vi "Axsun_subvi.vi"(10 "Clock delay":u32, 11 "Action":T1) -> (0 "error out":errorcluster, 3 "output cluster":T2)   [LabVIEW 2018]
uses:
  cluster_Axsun.ctl
  Action_Axsun.ctl
  C:/Users/BoasLab/Documents/stephan/Axsun control/AxsunOCTControl.dll
  AxsunOCTControl.dll
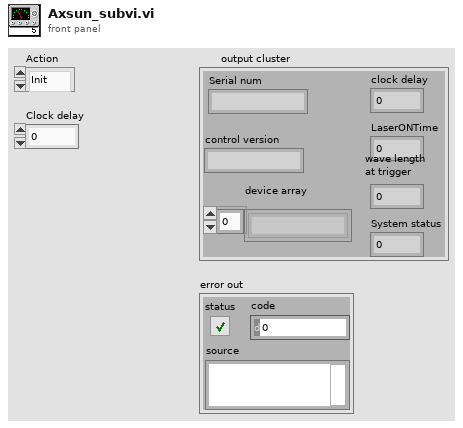
[diagram p1: front panel]
types:
  T1 = typedef "Action_Axsun.ctl" = enum16{"Init", "Stop", "Source current ON", "Source current OFF", "Laser ON", "Laser OFF", "GetLaserOnTime", "Clock delay"}
  T2 = typedef "cluster_Axsun.ctl" = cluster{"device array":string[], "control version":string, "Serial num":string, "LaserONTime":i32, "wave length\nat trigger":dbl, "System status":dbl, "clock delay":u32}
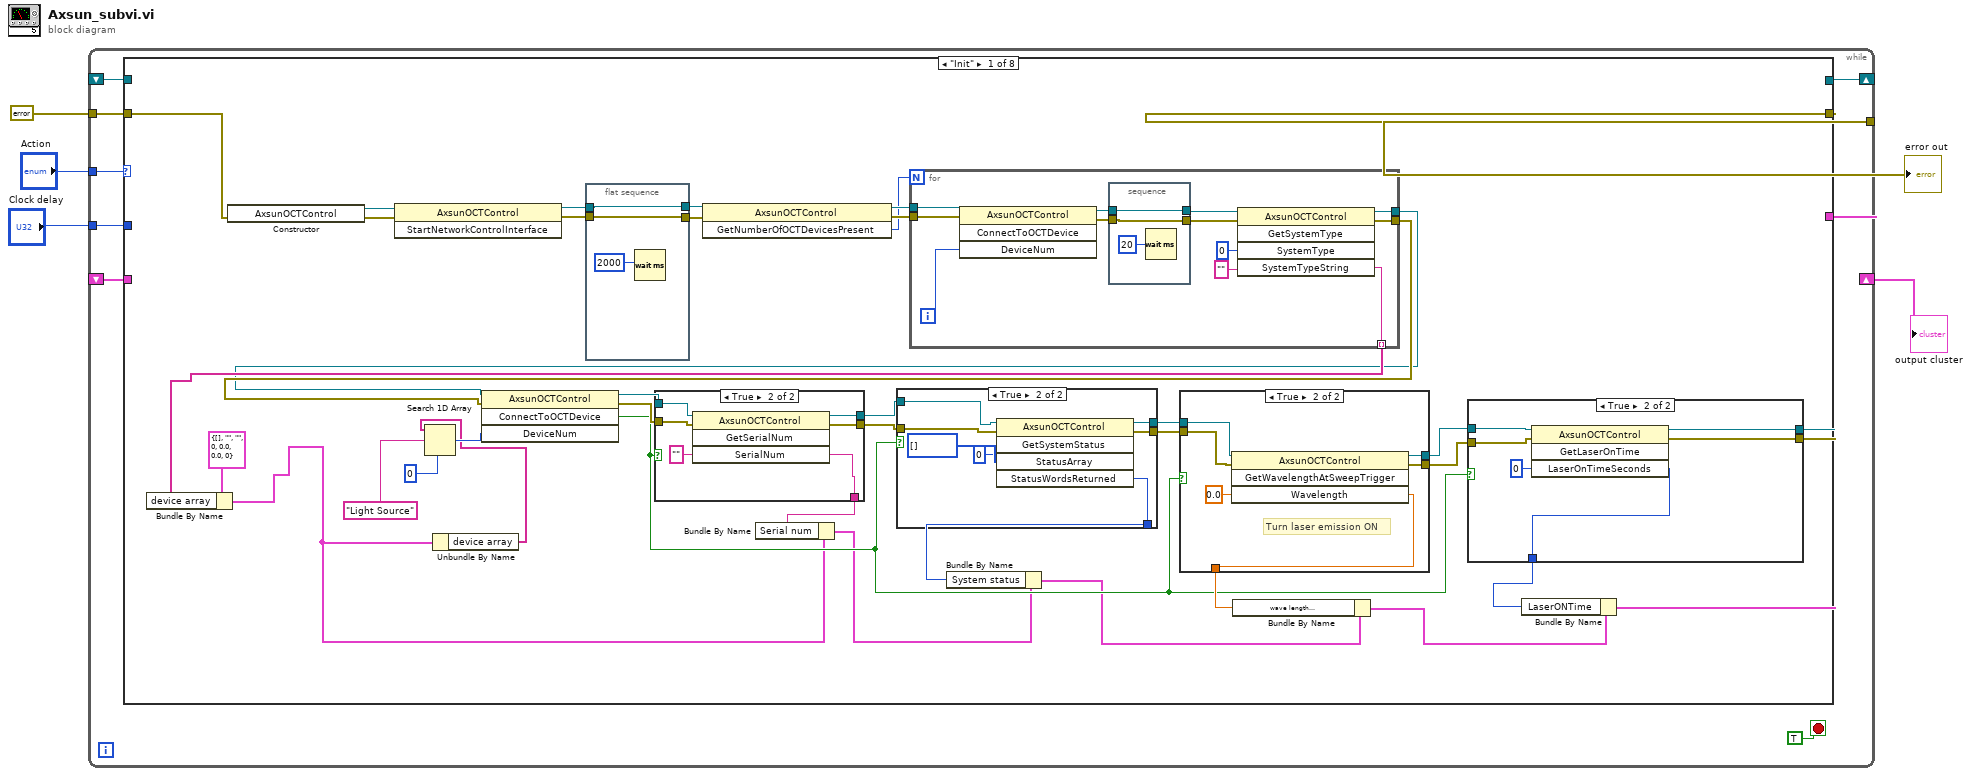
[diagram p0: block diagram]
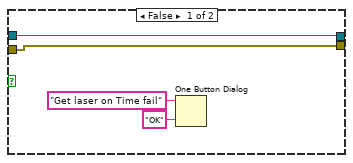
[diagram p2: hidden frame]
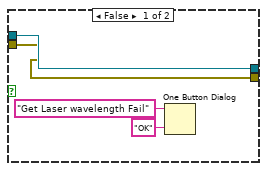
[diagram p3: hidden frame]
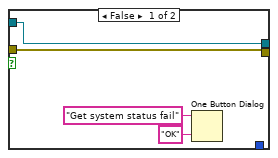
[diagram p4: hidden frame]
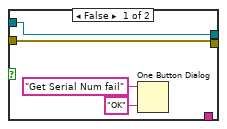
[diagram p5: hidden frame]
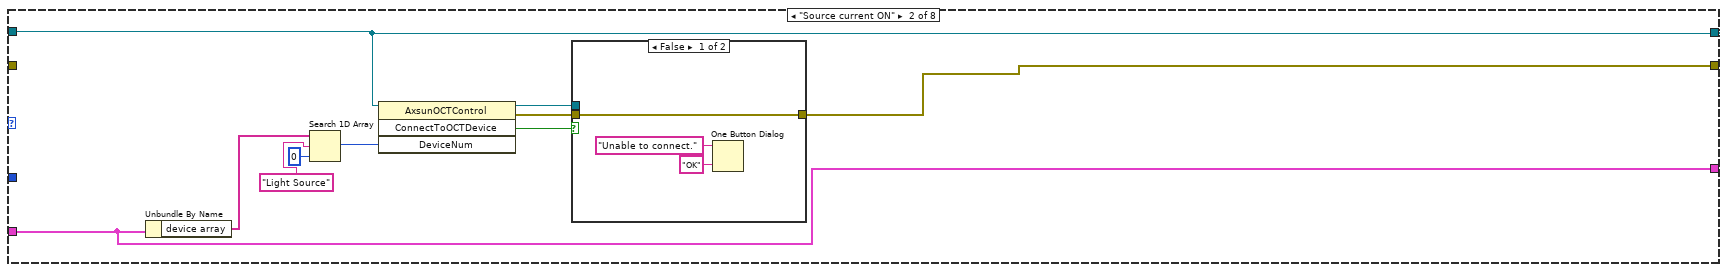
[diagram p6: hidden frame]
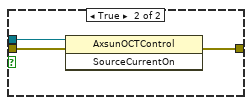
[diagram p7: hidden frame]
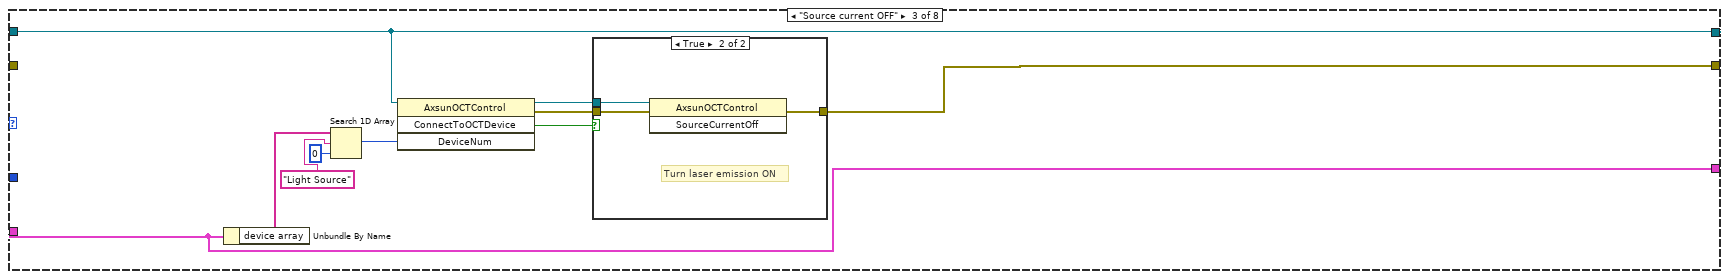
[diagram p8: hidden frame]
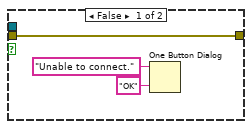
[diagram p9: hidden frame]
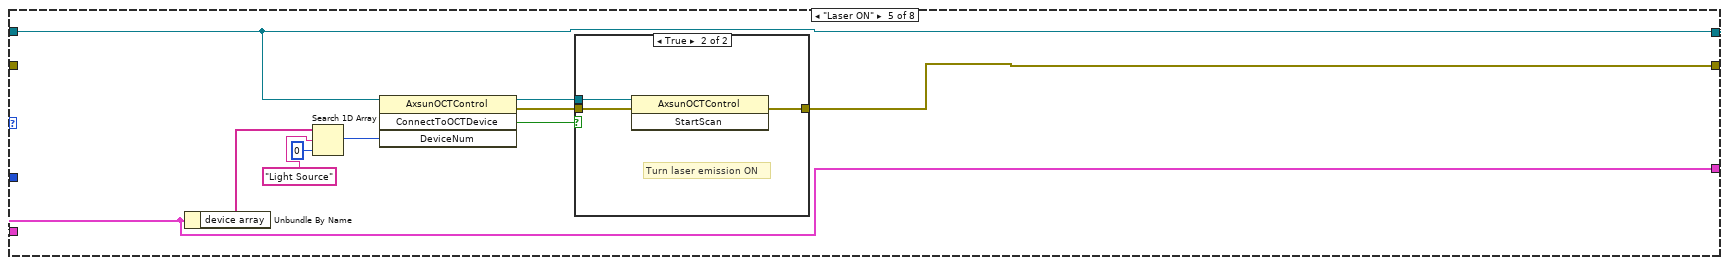
[diagram p11: hidden frame]
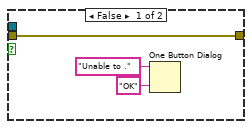
[diagram p12: hidden frame]
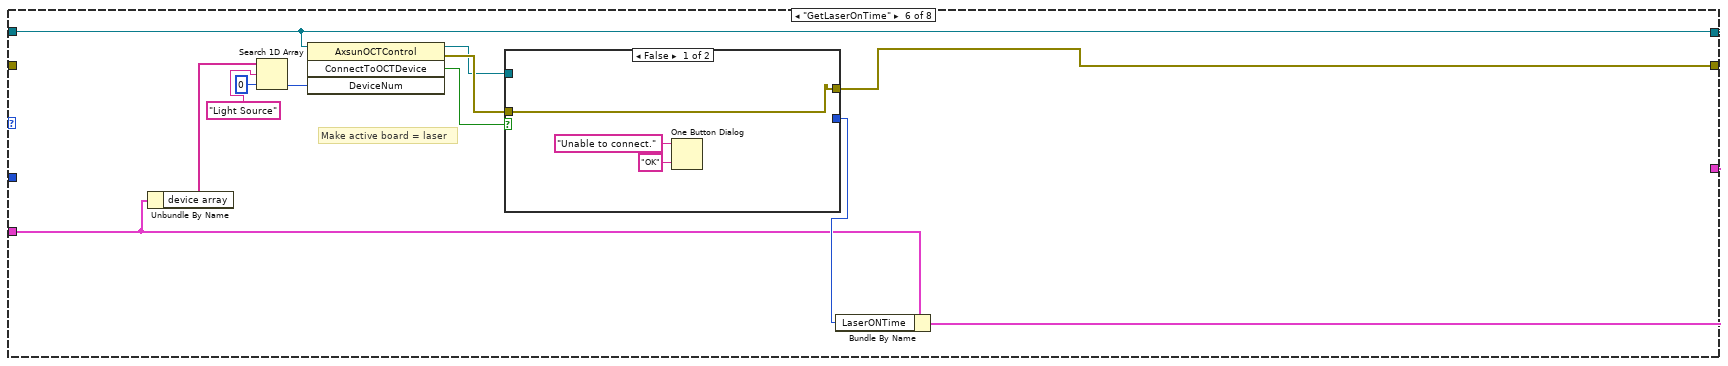
[diagram p13: hidden frame]
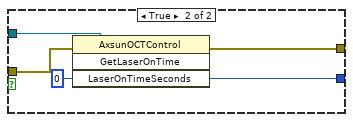
[diagram p14: hidden frame]
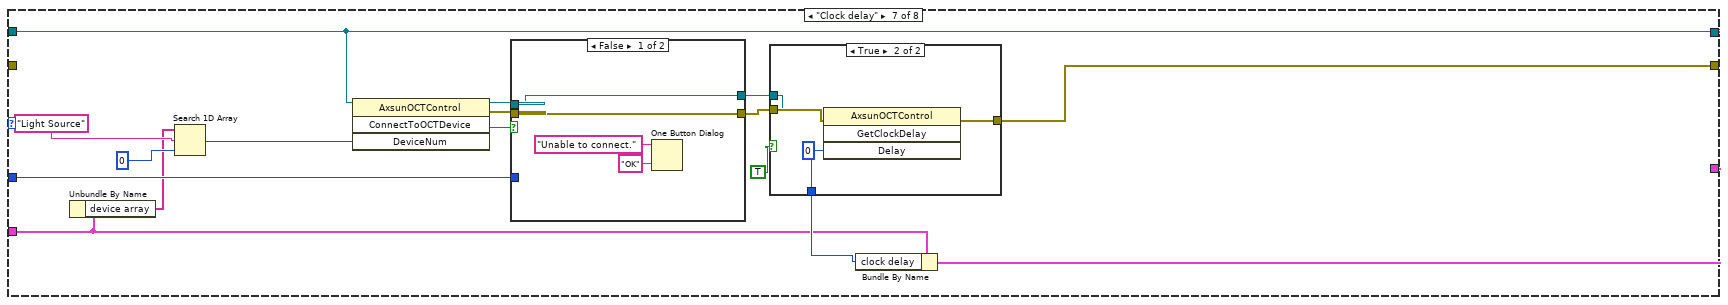
[diagram p15: hidden frame]
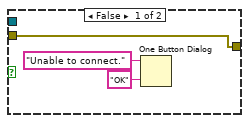
[diagram p16: hidden frame]
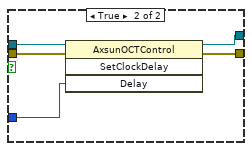
[diagram p17: hidden frame]
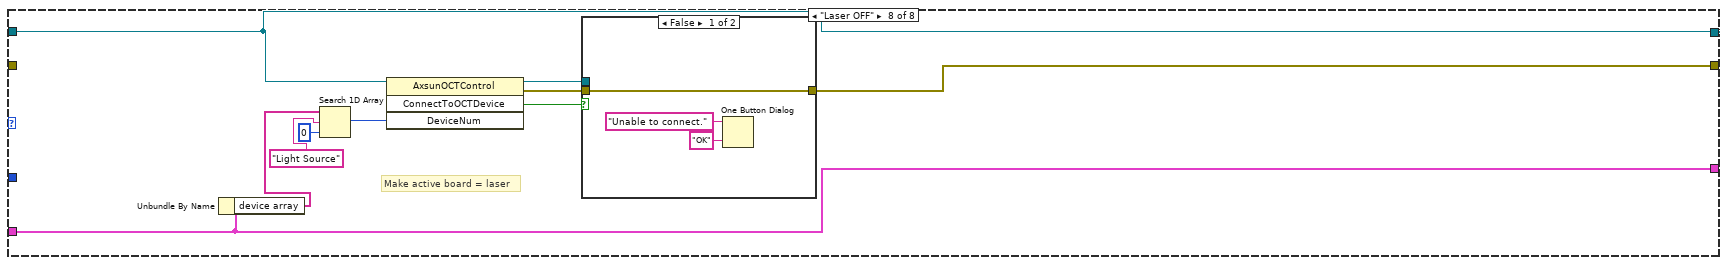
[diagram p18: hidden frame]
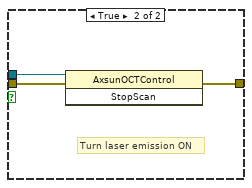
[diagram p19: hidden frame]
diagram:
  n1 = while {
    shift-right: [w11] -> _
    shift-left: _ -> [w12]
    shift-right: [w8] -> w2
    shift-left: _ -> [w14]
    tunnel: [w13] -> w4
    tunnel: "Clock delay" -> [w10]
    tunnel: "Action" -> [w9]
    tunnel: errorcluster {"status"=FALSE, "code"=0, "source"=""} ("error in (no error)") -> [w6]
    stop <- TRUE ("stop") stop-if-true
    n2 = case shown="\"Init\"" w9 {
      tunnel: [w28 w116 w132 _ w150 w168 w190 w219] -> w13
      tunnel: [w24 w113 w129 w144 w147 w163 w187 w216] -> w8
      tunnel: w14 -> [_ w113 w129 w144 w147 w166 w185 w216]
      tunnel: [w29 w112 w128 w145 w146 w162 w183 w215] -> w11
      tunnel: w12 -> [_ w112 w128 w145 w146 w162 w183 w215]
      tunnel: w10 -> [_ _ _ _ _ _ w188 _]
      tunnel: w6 -> [w15 _ _ _ _ _ _ _]
      frame "Init" {
        n3 = constructor class="AxsunOCTControl"(error in=w15) -> (reference out=w52:refnum<k24>, error out=w51:errorcluster)  [unwired: 2 in, 1 out]
        n4 = invoke class="AxsunOCTControl" method="StartNetworkControlInterface"(reference=w52, error in=w51) -> (reference out=w50:refnum<k24>, error out=w48:errorcluster)  [unwired: 1 in, 1 out]
        n5 = flat-sequence {
          tunnel: w50 -> [w110]
          tunnel: [w110] -> w49
          tunnel: [w109] -> w47
          tunnel: w48 -> [w109]
          frame #0 {
            n6 = Wait (ms)(milliseconds to wait=2000) -> ()  [unwired: 1 out]
          }
        }
        n7 = invoke class="AxsunOCTControl" method="GetNumberOfOCTDevicesPresent"(reference=w49, error in=w47) -> (reference out=w46:refnum<k24>, error out=w45:errorcluster, "GetNumberOfOCTDevicesPresent"=w19:i32)  [unwired: 1 in]
        n8 = for {
          N: w19 -> [_]
          tunnel: [w98] -> w18
          tunnel: [w97] -> w17
          tunnel: w46 -> [w96]
          tunnel: w45 -> [w95]
          tunnel: [w94] -> w23 mode=indexing
          i -> [w99]
          n9 = invoke class="AxsunOCTControl" method="ConnectToOCTDevice"(reference=w96, error in=w95, "DeviceNum"=w99) -> (reference out=w103:refnum<k24>, error out=w102:errorcluster)  [unwired: 1 in, 2 out]
          n10 = stacked-sequence {
            tunnel: w103 -> [w108]
            tunnel: [w108] -> w101
            tunnel: w102 -> [w107]
            tunnel: [w107] -> w100
            frame #0 {
              n11 = Wait (ms)(milliseconds to wait=u32 20) -> ()  [unwired: 1 out]
            }
          }
          n12 = invoke class="AxsunOCTControl" method="GetSystemType"(reference=w101, error in=w100, "SystemType"=u32 0, "SystemTypeString"="") -> (reference out=w97:refnum<k24>, error out=w98:errorcluster, "SystemTypeString"=w94:string)  [unwired: 1 in, 2 out]
        }
        n13 = Bundle By Name(cluster=T2 {"device array"=[], "control version"="", "Serial num"="", "LaserONTime"=0, "wave length\nat trigger"=0.0, "System status"=0.0, "clock delay"=0} ("output cluster"), "device array"=w23) -> (w16:T2)
        n14 = Unbundle By Name(w16) -> ("device array"=w21:string[])
        n15 = Search 1D Array(1D array=w21, element="Light Source", start index (0)=0) -> (index of element=w42:i32)
        n16 = invoke class="AxsunOCTControl" method="ConnectToOCTDevice"(reference=w17, error in=w18, "DeviceNum"=w42) -> (reference out=w41:refnum<k24>, error out=w40:errorcluster, "ConnectToOCTDevice"=w31:bool)  [unwired: 1 in, 1 out]
        n17 = case shown="True" w31 {
          tunnel: [w84 w93] -> w37
          tunnel: [_ w91] -> w43
          tunnel: w41 -> [w85 w90]
          tunnel: w40 -> [w84 w89]
          tunnel: [w85 w88] -> w38
          frame False {
            n18 = One Button Dialog(message="Get Serial Num fail", button name ("OK")="OK") -> ()  [unwired: 1 out]
          }
          frame True {
            n19 = invoke class="AxsunOCTControl" method="GetSerialNum"(reference=w90, error in=w89, "SerialNum"="") -> (reference out=w88:refnum<k24>, error out=w93:errorcluster, "SerialNum"=w91:string)  [unwired: 1 in, 1 out]
          }
        }
        n20 = Bundle By Name(cluster=w16, "Serial num"=w43) -> (w27:T2)
        n21 = case shown="True" w31 {
          tunnel: [_ w81] -> w39
          tunnel: w38 -> [w74 w80]
          tunnel: w37 -> [w73 w79]
          tunnel: [w74 w78] -> w36
          tunnel: [w73 w77] -> w35
          frame False {
            n22 = One Button Dialog(message="Get system status fail", button name ("OK")="OK") -> ()  [unwired: 1 out]
          }
          frame True {
            n23 = invoke class="AxsunOCTControl" method="GetSystemStatus"(reference=w80, error in=w79, "StatusArray"=u32[] [], "StatusWordsReturned"=u32 0) -> (reference out=w78:refnum<k24>, error out=w77:errorcluster, "StatusWordsReturned"=w81:u32)  [unwired: 1 in, 2 out]
          }
        }
        n24 = Bundle By Name(cluster=w27, "System status"=w39) -> (w26:T2)
        n25 = case shown="True" w31 {
          tunnel: [w63 w72] -> w32
          tunnel: w36 -> [w64 w70]
          tunnel: w35 -> [w63 w69]
          tunnel: [_ w68] -> w34
          tunnel: [w64 w67] -> w33
          frame False {
            n26 = One Button Dialog(message="Get Laser wavelength Fail", button name ("OK")="OK") -> ()  [unwired: 1 out]
          }
          frame True {
            # "Turn laser emission ON"
            n27 = invoke class="AxsunOCTControl" method="GetWavelengthAtSweepTrigger"(reference=w70, error in=w69, "Wavelength"=0.0) -> (reference out=w67:refnum<k24>, error out=w72:errorcluster, "Wavelength"=w68:dbl)  [unwired: 1 in, 1 out]
          }
        }
        n28 = Bundle By Name(cluster=w26, "wave length\nat trigger"=w34) -> (w25:T2)
        n29 = case shown="True" w31 {
          tunnel: [w53 w62] -> w28
          tunnel: w33 -> [w54 w60]
          tunnel: w32 -> [w53 w59]
          tunnel: [_ w58] -> w30
          tunnel: [w54 w57] -> w29
          frame False {
            n30 = One Button Dialog(message="Get laser on Time fail", button name ("OK")="OK") -> ()  [unwired: 1 out]
          }
          frame True {
            n31 = invoke class="AxsunOCTControl" method="GetLaserOnTime"(reference=w60, error in=w59, "LaserOnTimeSeconds"=u32 0) -> (reference out=w57:refnum<k24>, error out=w62:errorcluster, "LaserOnTimeSeconds"=w58:u32)  [unwired: 1 in, 1 out]
          }
        }
        n32 = Bundle By Name(cluster=w25, "LaserONTime"=w30) -> (w24:T2)
      }
      frame "Source current ON" {
        n33 = Unbundle By Name(w113) -> ("device array"=w115:string[])
        n34 = Search 1D Array(1D array=w115, element="Light Source", start index (0)=0) -> (index of element=w120:i32)
        n35 = invoke class="AxsunOCTControl" method="ConnectToOCTDevice"(reference=w112, "DeviceNum"=w120) -> (reference out=w119:refnum<k24>, error out=w118:errorcluster, "ConnectToOCTDevice"=w117:bool)  [unwired: 2 in, 1 out]
        n36 = case shown="False" w117 {
          tunnel: w119 -> [_ w127]
          tunnel: w118 -> [w124 w126]
          tunnel: [w124 w125] -> w116
          frame False {
            n37 = One Button Dialog(message="Unable to connect.", button name ("OK")="OK") -> ()  [unwired: 1 out]
          }
          frame True {
            n38 = invoke class="AxsunOCTControl" method="SourceCurrentOn"(reference=w127, error in=w126) -> (error out=w125:errorcluster)  [unwired: 1 in, 2 out]
          }
        }
      }
      frame "Source current OFF" {
        n39 = Unbundle By Name(w129) -> ("device array"=w131:string[])
        n40 = Search 1D Array(1D array=w131, element="Light Source", start index (0)=0) -> (index of element=w136:i32)
        n41 = invoke class="AxsunOCTControl" method="ConnectToOCTDevice"(reference=w128, "DeviceNum"=w136) -> (reference out=w135:refnum<k24>, error out=w134:errorcluster, "ConnectToOCTDevice"=w133:bool)  [unwired: 2 in, 1 out]
        n42 = case shown="True" w133 {
          tunnel: w135 -> [_ w143]
          tunnel: w134 -> [w140 w142]
          tunnel: [w140 w141] -> w132
          frame False {
            n43 = One Button Dialog(message="Unable to connect.", button name ("OK")="OK") -> ()  [unwired: 1 out]
          }
          frame True {
            # "Turn laser emission ON"
            n44 = invoke class="AxsunOCTControl" method="SourceCurrentOff"(reference=w143, error in=w142) -> (error out=w141:errorcluster)  [unwired: 1 in, 2 out]
          }
        }
      }
      frame Default {
      }
      frame "Laser ON" {
        n45 = Unbundle By Name(w147) -> ("device array"=w149:string[])
        n46 = Search 1D Array(1D array=w149, element="Light Source", start index (0)=0) -> (index of element=w154:i32)
        n47 = invoke class="AxsunOCTControl" method="ConnectToOCTDevice"(reference=w146, "DeviceNum"=w154) -> (reference out=w153:refnum<k24>, error out=w152:errorcluster, "ConnectToOCTDevice"=w151:bool)  [unwired: 2 in, 1 out]
        n48 = case shown="True" w151 {
          tunnel: w153 -> [_ w161]
          tunnel: w152 -> [w158 w160]
          tunnel: [w158 w159] -> w150
          frame False {
            n49 = One Button Dialog(message="Unable to .", button name ("OK")="OK") -> ()  [unwired: 1 out]
          }
          frame True {
            # "Turn laser emission ON"
            n50 = invoke class="AxsunOCTControl" method="StartScan"(reference=w161, error in=w160) -> (error out=w159:errorcluster)  [unwired: 1 in, 2 out]
          }
        }
      }
      frame "GetLaserOnTime" {
        # "Make active board = laser"
        n51 = Unbundle By Name(w166) -> ("device array"=w165:string[])
        n52 = Search 1D Array(1D array=w165, element="Light Source", start index (0)=0) -> (index of element=w173:i32)
        n53 = invoke class="AxsunOCTControl" method="ConnectToOCTDevice"(reference=w162, "DeviceNum"=w173) -> (reference out=w170:refnum<k24>, error out=w171:errorcluster, "ConnectToOCTDevice"=w169:bool)  [unwired: 2 in, 1 out]
        n54 = case shown="False" w169 {
          tunnel: w171 -> [w176 w180]
          tunnel: w170 -> [_ w181]
          tunnel: [w176 w179] -> w168
          tunnel: [_ w177] -> w167
          frame False {
            n55 = One Button Dialog(message="Unable to connect.", button name ("OK")="OK") -> ()  [unwired: 1 out]
          }
          frame True {
            n56 = invoke class="AxsunOCTControl" method="GetLaserOnTime"(reference=w181, error in=w180, "LaserOnTimeSeconds"=u32 0) -> (error out=w179:errorcluster, "LaserOnTimeSeconds"=w177:u32)  [unwired: 1 in, 2 out]
          }
        }
        n57 = Bundle By Name(cluster=w166, "LaserONTime"=w167) -> (w163:T2)
      }
      frame "Clock delay" {
        n58 = Unbundle By Name(w185) -> ("device array"=w184:string[])
        n59 = Search 1D Array(1D array=w184, element="Light Source", start index (0)=0) -> (index of element=w196:i32)
        n60 = invoke class="AxsunOCTControl" method="ConnectToOCTDevice"(reference=w183, "DeviceNum"=w196) -> (reference out=w195:refnum<k24>, error out=w194:errorcluster, "ConnectToOCTDevice"=w193:bool)  [unwired: 2 in, 1 out]
        n61 = case shown="False" w193 {
          tunnel: w195 -> [w206 w214]
          tunnel: w194 -> [w209 w213]
          tunnel: [w209 w212] -> w192
          tunnel: w188 -> [_ w211]
          tunnel: [w206 w210] -> w182
          frame False {
            n62 = One Button Dialog(message="Unable to connect.", button name ("OK")="OK") -> ()  [unwired: 1 out]
          }
          frame True {
            n63 = invoke class="AxsunOCTControl" method="SetClockDelay"(reference=w214, error in=w213, "Delay"=w211) -> (reference out=w210:refnum<k24>, error out=w212:errorcluster)  [unwired: 1 in, 2 out]
          }
        }
        n64 = case shown="True" TRUE {
          tunnel: w192 -> [w200 w205]
          tunnel: [w200 w204] -> w190
          tunnel: [_ w202] -> w189
          tunnel: w182 -> [_ w201]
          frame False {
            n65 = One Button Dialog(message="Unable to connect.", button name ("OK")="OK") -> ()  [unwired: 1 out]
          }
          frame True {
            n66 = invoke class="AxsunOCTControl" method="GetClockDelay"(reference=w201, error in=w205, "Delay"=u32 0) -> (error out=w204:errorcluster, "Delay"=w202:u32)  [unwired: 1 in, 2 out]
          }
        }
        n67 = Bundle By Name(cluster=w185, "clock delay"=w189) -> (w187:T2)
      }
      frame "Laser OFF" {
        # "Make active board = laser"
        n68 = Unbundle By Name(w216) -> ("device array"=w218:string[])
        n69 = Search 1D Array(1D array=w218, element="Light Source", start index (0)=0) -> (index of element=w223:i32)
        n70 = invoke class="AxsunOCTControl" method="ConnectToOCTDevice"(reference=w215, "DeviceNum"=w223) -> (reference out=w222:refnum<k24>, error out=w221:errorcluster, "ConnectToOCTDevice"=w220:bool)  [unwired: 2 in, 1 out]
        n71 = case shown="False" w220 {
          tunnel: w222 -> [_ w230]
          tunnel: w221 -> [w227 w229]
          tunnel: [w227 w228] -> w219
          frame False {
            n72 = One Button Dialog(message="Unable to connect.", button name ("OK")="OK") -> ()  [unwired: 1 out]
          }
          frame True {
            # "Turn laser emission ON"
            n73 = invoke class="AxsunOCTControl" method="StopScan"(reference=w230, error in=w229) -> (error out=w228:errorcluster)  [unwired: 1 in, 2 out]
          }
        }
      }
    }
  }
  "output cluster" <- w2
  "error out" <- w4
